vi "do-measurementSD.vi"(6 "Real delay time, ps":dbl, 7 "File":path, 8 "error in (no error)":errorcluster, 9 "Cluster in":T1={"error"=refnum, "RT exp"=refnum, "# current"=refnum, "Start measurement"=refnum, "GRAPH EXPERIMENTAL DATA"=refnum, "DelaysTab"=enum."Table", "slider"=refnum, "aq contol"=enum."fixed", "RDT, ps"=refnum, "table delays"=[-500.0, -400.0, -0.0, 100.0, 250.0, 350.0], "notifier mesure in"=refnum, "Measure finished"=refnum, "Measure event"=refnum, "Laser shutter task"="", "minmaxOD"={"ODmin"=0.0, "ODmax"=0.0}}, 11 "Experiment in":refnum<class "Experiment.lvclass">) -> (0 "error out":errorcluster, 2 "graph data":dbl[][](array[numeric]), 3 "Experiment out":refnum<class "Experiment.lvclass">)   [LabVIEW 2015]
uses:
  Classes/Experiment.lvclass
  controls/clustercontrols-measerument.ctl
  globalVarSD.vi
panel:
  out "Numérique":i32
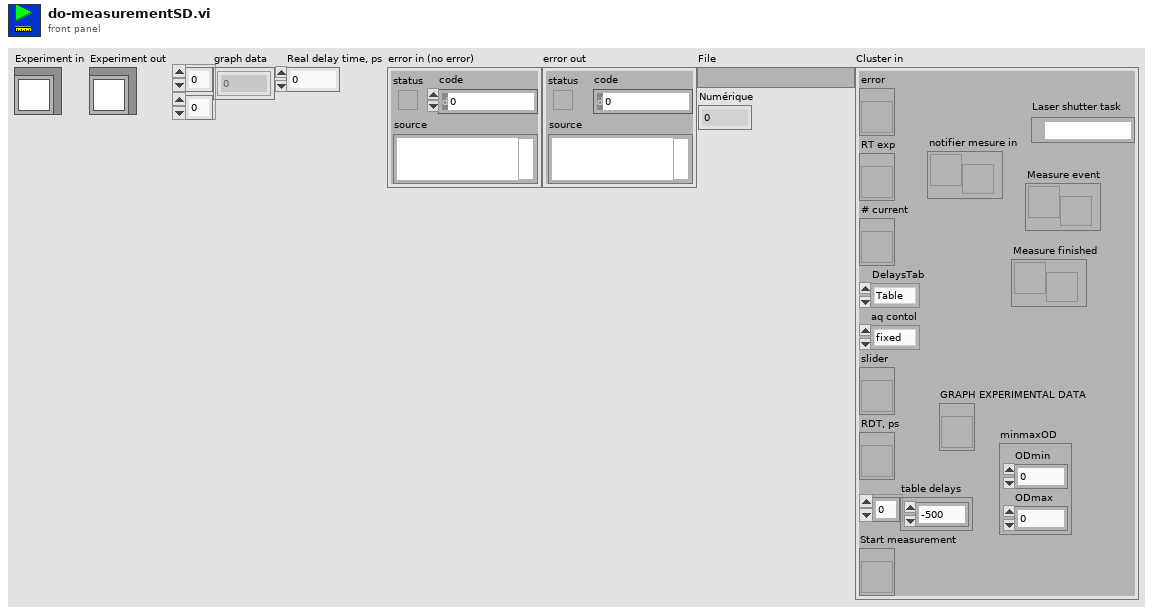
[diagram p1: front panel]
types:
  T1 = typedef "clustercontrols-measerument.ctl" = cluster{"error":refnum<vi>, "RT exp":refnum<vi>, "# current":refnum<vi>, "Start measurement":refnum<vi>, "GRAPH EXPERIMENTAL DATA":refnum<vi>, "DelaysTab":enum32{"Mode Normale", "Table"}, "slider":refnum<vi>, "aq contol":enum32{"fixed", "automatic", "fixed-auto"}, "RDT, ps":refnum<vi>, "table delays":dbl[], "notifier mesure in":refnum<notifier>, "Measure finished":refnum<user-event>, "Measure event":refnum<user-event>, "Laser shutter task":refnum<k21>, "minmaxOD":cluster{"ODmin":dbl, "ODmax":dbl}}
  T2 = typedef "data-cluster.ctl" = cluster{"BG":i32[], "Ie":i32[], "I0":i32[]}[]
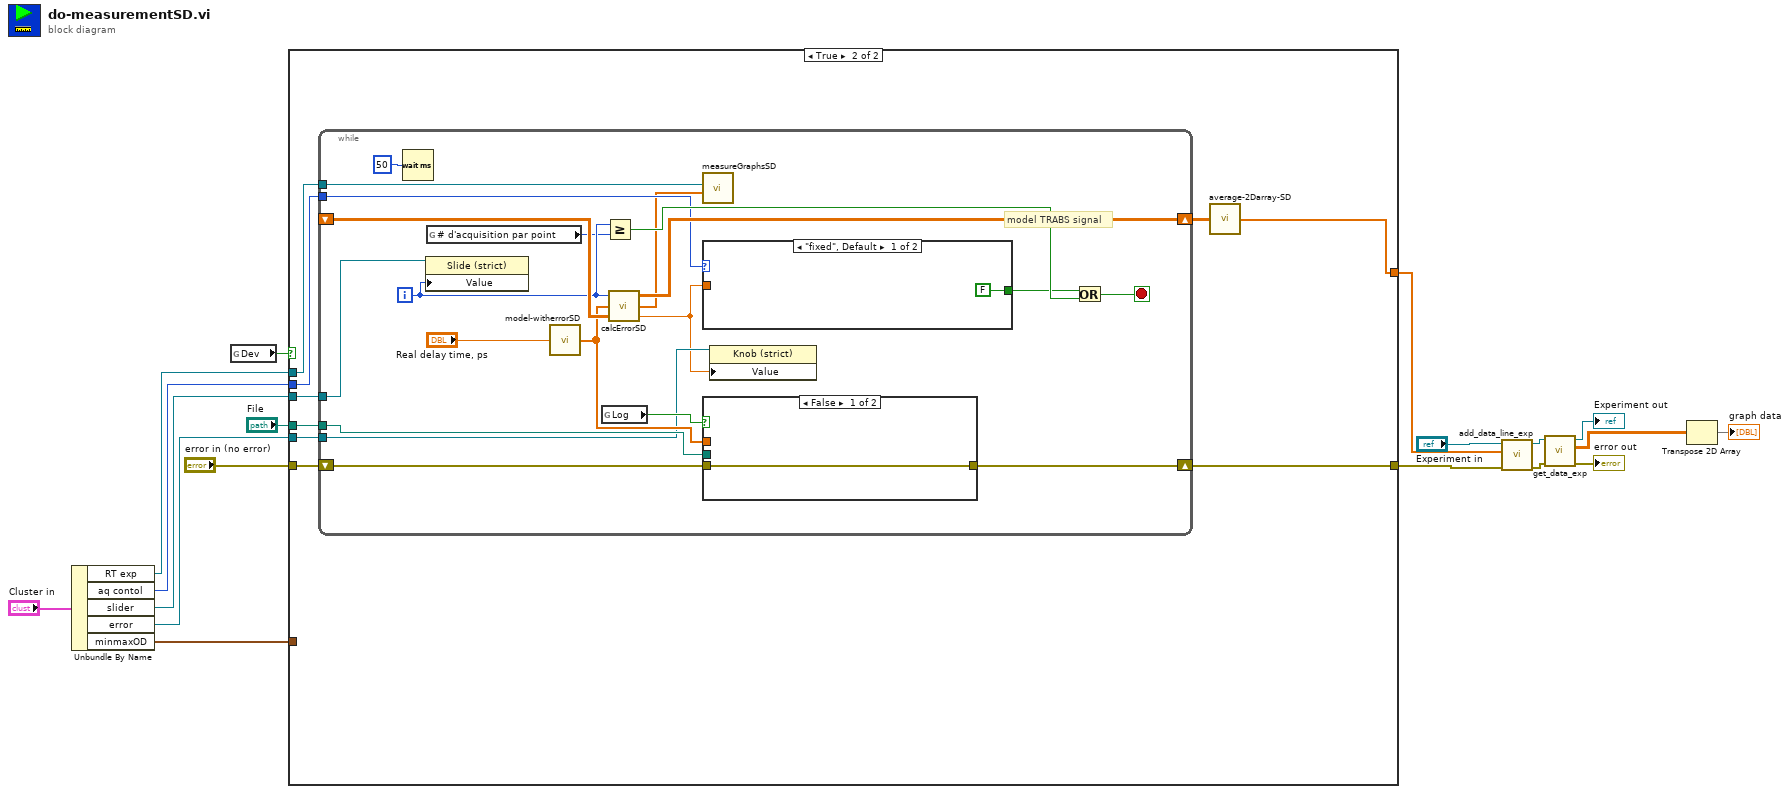
[diagram p0: block diagram]
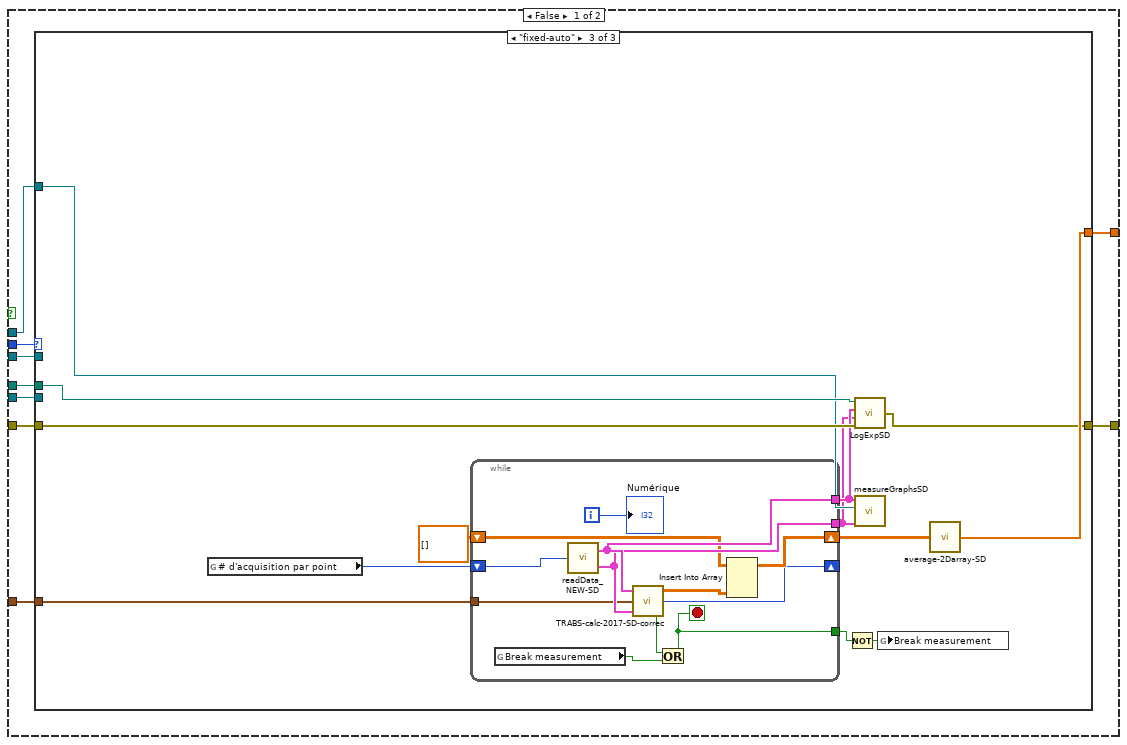
[diagram p2: hidden frame]
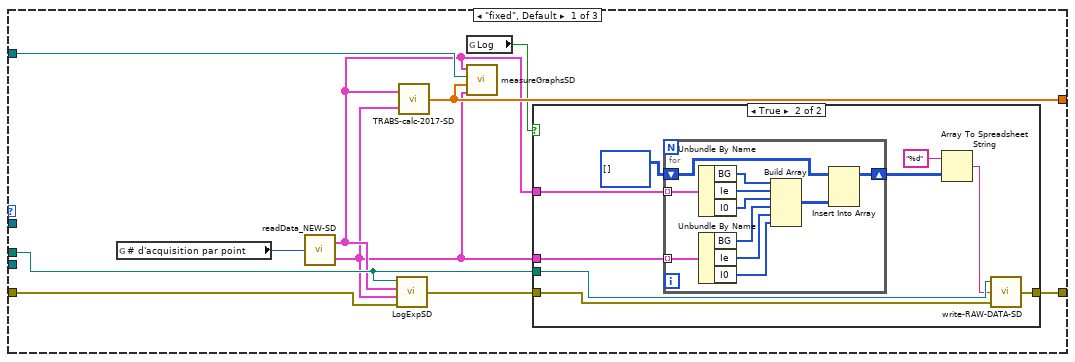
[diagram p3: hidden frame]
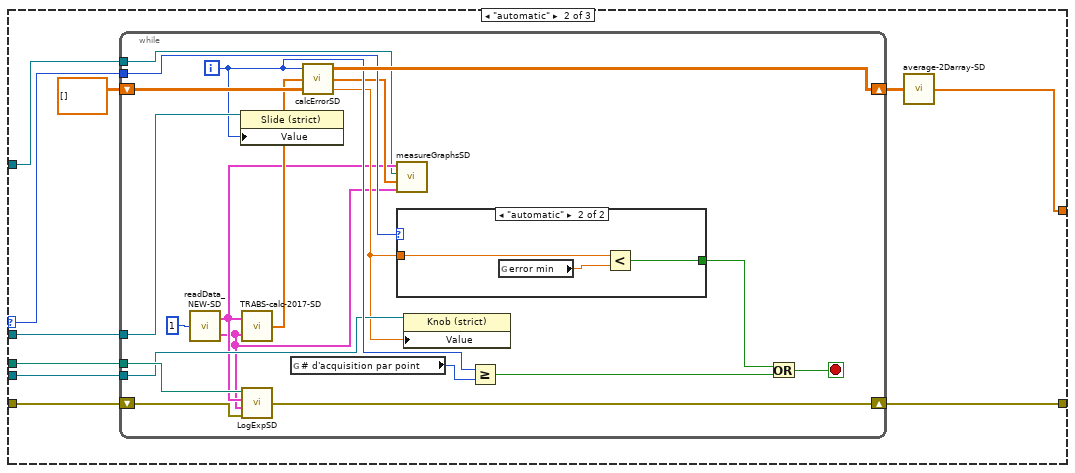
[diagram p5: hidden frame]
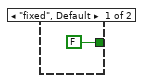
[diagram p6: hidden frame]
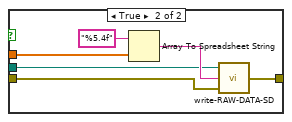
[diagram p7: hidden frame]
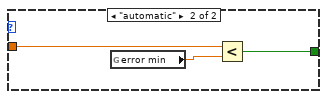
[diagram p8: hidden frame]
diagram:
  n1 = Unbundle By Name("Cluster in") -> ("RT exp"=w3:refnum<vi>, "aq contol"=w2:enum32{"fixed", "automatic", "fixed-auto"}, "slider"=w5:refnum<vi>, "error"=w4:refnum<vi>, "minmaxOD"=w1:cluster{"ODmin":dbl, "ODmax":dbl})
  n2 = global read "globalVarSD.vi" "Dev"() -> (w12:bool)
  n3 = case shown="True" w12 {
    tunnel: w2 -> [w27 w126]
    tunnel: w5 -> [w23 w125]
    tunnel: w4 -> [w22 w124]
    tunnel: "File" -> [w26 w123]
    tunnel: "error in (no error)" -> [w25 w122]
    tunnel: [w24 w121] -> w8
    tunnel: [w21 w119] -> w7
    tunnel: w3 -> [w20 w118]
    tunnel: w1 -> [w19 _]
    frame False {
      n4 = case shown="\"fixed-auto\"" w27 {
        selector: w27 -> [_ w66 _]
        tunnel: [w35 w67 w105] -> w21
        tunnel: w26 -> [w30 w65 w104]
        tunnel: w25 -> [w36 w64 w103]
        tunnel: [w31 w63 w102] -> w24
        tunnel: w23 -> [_ w62 _]
        tunnel: w22 -> [_ w61 _]
        tunnel: w20 -> [w34 w60 w101]
        tunnel: w19 -> [_ _ w100]
        frame "fixed", Default {
          n5 = global read "globalVarSD.vi" "# d'acquisition par point"() -> (w37:u32)
          n6 = call "readData_NEW-SD.vi"("number of aq"=w37) -> ("I channel seq"=w29:T2, "II channel seq"=w28:T2)
          n7 = call "LogExpSD.vi"("error in (no error)"=w36, "II channel seq"=w28, "I channel seq"=w29, "File"=w30) -> ("error out"=w32:errorcluster)
          n8 = call "TRABS-calc-2017-SD.vi"("II channel seq"=w28, "I channel seq"=w29) -> ("TRABS"=w35:dbl[])
          n9 = global read "globalVarSD.vi" "Log"() -> (w33:bool)
          n10 = call "measureGraphsSD.vi"("II channel seq"=w28, "OD averaged"=w35, "Real Time Experiment"=w34, "I channel seq"=w29) -> ()
          n11 = case shown="True" w33 {
            tunnel: [w38 w46] -> w31
            tunnel: w32 -> [w38 w45]
            tunnel: w30 -> [_ w47]
            tunnel: w29 -> [_ w44]
            tunnel: w28 -> [_ w43]
            frame False {
            }
            frame True {
              n12 = for {
                tunnel: w44 -> [w58] mode=indexing
                tunnel: w43 -> [w57] mode=indexing
                shift-right: [w48] -> w39
                shift-left: i32[][] [] -> [w49]
                n13 = Unbundle By Name(w58) -> ("BG"=w56:i32[], "Ie"=w55:i32[], "I0"=w54:i32[])
                n14 = Unbundle By Name(w57) -> ("BG"=w53:i32[], "Ie"=w52:i32[], "I0"=w51:i32[])
                n15 = Build Array(w56, w55, w54, w53, w52, w51) -> (w50:i32[][])
                n16 = Insert Into Array(array=w49, new element=w50) -> (w48:i32[][])  [unwired: 2 in]
              }
              n17 = Array To Spreadsheet String(array=w39, 3:"%d" ("format string")) -> (spreadsheet string=w40:string)  [unwired: 1 in]
              n18 = call "write-RAW-DATA-SD.vi"("error in (no error)"=w45, "Text"=w40, "File"=w47) -> ("error out"=w46:errorcluster)
            }
          }
        }
        frame "automatic" {
          n19 = while {
            shift-right: [w88] -> w68
            shift-left: dbl[][] [] ("Array out") -> [w87]
            tunnel: w66 -> [w82]
            tunnel: w65 -> [w81]
            shift-right: [w80] -> w63
            shift-left: w64 -> [w79]
            tunnel: w62 -> [w76]
            tunnel: w61 -> [w74]
            tunnel: w60 -> [w69]
            i -> [w75]
            stop <- w85 stop-if-true
            n20 = call "readData_NEW-SD.vi"("number of aq"=1) -> ("I channel seq"=w71:T2, "II channel seq"=w70:T2)
            n21 = property class="Slide (strict)"(reference=w76, "Value"=w75) -> ()  [unwired: 1 in, 2 out]
            n22 = call "TRABS-calc-2017-SD.vi"("II channel seq"=w70, "I channel seq"=w71) -> ("TRABS"=w78:dbl[])
            n23 = call "LogExpSD.vi"("error in (no error)"=w79, "II channel seq"=w70, "I channel seq"=w71, "File"=w81) -> ("error out"=w80:errorcluster)
            n24 = global read "globalVarSD.vi" "# d'acquisition par point"() -> (w77:u32)
            n25 = call "calcErrorSD.vi"("array of OD"=w87, "OD"=w78, "Numeric in"=w75) -> ("error out"=w73:dbl, "average out"=w72:dbl[], "Array out"=w88:dbl[][])
            n26 = call "measureGraphsSD.vi"("II channel seq"=w70, "OD averaged"=w72, "Real Time Experiment"=w69, "I channel seq"=w71) -> ()
            n27 = case shown="\"automatic\"" w82 {
              tunnel: w73 -> [_ w92]
              tunnel: [FALSE w91] -> w86
              frame "fixed", Default {
              }
              frame "automatic" {
                n28 = global read "globalVarSD.vi" "error min"() -> (w90:dbl)
                n29 = Less?(x=w92, y=w90) -> (x < y?=w91:bool)
              }
            }
            n30 = property class="Knob (strict)"(reference=w74, "Value"=w73) -> ()  [unwired: 1 in, 2 out]
            n31 = Greater Or Equal?(x=w75, y=w77) -> (x >= y?=w83:bool)
            n32 = Or(x=w86, y=w83) -> (x .or. y?=w85:bool)
          }
          n33 = call "average-2Darray-SD.vi"("2D array"=w68) -> ("out array"=w67:dbl[])
        }
        frame "fixed-auto" {
          n34 = global read "globalVarSD.vi" "# d'acquisition par point"() -> (w96:u32)
          n35 = while {
            tunnel: [w117] -> w98
            tunnel: [w116] -> w97
            tunnel: w100 -> [w115]
            shift-right: [w109] -> _
            shift-left: w96 -> [w113]
            shift-right: [w111] -> w99
            shift-left: dbl[][] [] ("TRABS") -> [w112]
            tunnel: [w106] -> w94
            i -> [w114]
            stop <- w106 stop-if-true
            n36 = global read "globalVarSD.vi" "Break measurement"() -> (w107:bool)
            n37 = call "readData_NEW-SD.vi"("number of aq"=w113) -> ("I channel seq"=w117:T2, "II channel seq"=w116:T2)
            n38 = call "TRABS-calc-2017-SD-correc.vi"("II channel seq"=w116, "minmaxOD"=w115, "I channel seq"=w117) -> ("Finished"=w108:bool, "diffpoints"=w109:i32, "TRABS"=w110:dbl[][])
            n39 = Or(x=w108, y=w107) -> (x .or. y?=w106:bool)
            n40 = Insert Into Array(array=w112, new element=w110) -> (w111:dbl[][])  [unwired: 2 in]
            "Numérique" <- w114
          }
          n41 = Not(x=w94) -> (.not. x?=w93:bool)
          n42 = call "LogExpSD.vi"("error in (no error)"=w103, "II channel seq"=w97, "I channel seq"=w98, "File"=w104) -> ("error out"=w102:errorcluster)
          n43 = call "measureGraphsSD.vi"("II channel seq"=w97, "Real Time Experiment"=w101, "I channel seq"=w98) -> ()  [unwired: 1 in]
          n44 = global write "globalVarSD.vi" "Break measurement"(w93) -> ()
          n45 = call "average-2Darray-SD.vi"("2D array"=w99) -> ("out array"=w105:dbl[])
        }
      }
    }
    frame True {
      n46 = while {
        shift-right: [w143] -> w120
        shift-left: _ -> [w144]
        tunnel: w126 -> [w139]
        tunnel: w125 -> [w137]
        tunnel: w124 -> [w128]
        tunnel: w123 -> [w131]
        shift-right: [w134] -> w121
        shift-left: w122 -> [w133]
        tunnel: w118 -> [w129]
        i -> [w140]
        stop <- w142 stop-if-true
        # "model TRABS signal"
        n47 = Wait (ms)(milliseconds to wait=u32 50) -> ()  [unwired: 1 out]
        n48 = property class="Slide (strict)"(reference=w137, "Value"=w140) -> ()  [unwired: 1 in, 2 out]
        n49 = global read "globalVarSD.vi" "# d'acquisition par point"() -> (w136:u32)
        n50 = call "model-witherrorSD.vi"("Real delay time, ps"="Real delay time, ps") -> ("Array"=w132:dbl[])
        n51 = global read "globalVarSD.vi" "Log"() -> (w135:bool)
        n52 = Greater Or Equal?(x=w140, y=w136) -> (x >= y?=w141:bool)
        n53 = call "calcErrorSD.vi"("array of OD"=w144, "OD"=w132, "Numeric in"=w140) -> ("error out"=w127:dbl, "average out"=w130:dbl[], "Array out"=w143:dbl[][])
        n54 = call "measureGraphsSD.vi"("OD averaged"=w130, "Real Time Experiment"=w129) -> ()  [unwired: 2 in]
        n55 = case shown="\"fixed\", Default" w139 {
          tunnel: w127 -> [_ w157]
          tunnel: [FALSE w156] -> w138
          frame "fixed", Default {
          }
          frame "automatic" {
            n56 = global read "globalVarSD.vi" "error min"() -> (w155:dbl)
            n57 = Less?(x=w157, y=w155) -> (x < y?=w156:bool)
          }
        }
        n58 = case shown="False" w135 {
          tunnel: [w147 w151] -> w134
          tunnel: w133 -> [w147 w150]
          tunnel: w132 -> [_ w148]
          tunnel: w131 -> [_ w152]
          frame False {
          }
          frame True {
            n59 = Array To Spreadsheet String(array=w148, 3:"%5.4f" ("format string")) -> (spreadsheet string=w153:string)  [unwired: 1 in]
            n60 = call "write-RAW-DATA-SD.vi"("error in (no error)"=w150, "Text"=w153, "File"=w152) -> ("error out"=w151:errorcluster)
          }
        }
        n61 = property class="Knob (strict)"(reference=w128, "Value"=w127) -> ()  [unwired: 1 in, 2 out]
        n62 = Or(x=w138, y=w141) -> (x .or. y?=w142:bool)
      }
      n63 = call "average-2Darray-SD.vi"("2D array"=w120) -> ("out array"=w119:dbl[])
    }
  }
  n64 = call "add_data_line_exp.vi"("error in (no error)"=w8, "add Array"=w7, "Experiment.lvclass in"="Experiment in") -> ("error out"=w15:errorcluster, "Experiment.lvclass out"=w13:refnum<class "Experiment.lvclass">)  [unwired: 7 in]
  n65 = call "get_data_exp.vi"("error in (no error)"=w15, "Experiment.lvclass in"=w13) -> ("error out"=→"error out":errorcluster, "Data"=w17:dbl[][], "Experiment.lvclass out"=→"Experiment out":refnum<class "Experiment.lvclass">)  [unwired: 7 in]
  n66 = Transpose 2D Array(2D array=w17) -> (transposed array=→"graph data":dbl[][])
